vi "update file properties.vi"(4 "event name":string, 5 "mode":T2=enum."Rename Files", 6 "file format":T1(ring), 7 "scanner[]":string[](array[string]), 8 "error in":errorcluster, 9 "destination path":path, 10 "file path":path, 11 "File in":refnum<class "File.lvclass">) -> (0 "error out":errorcluster, 3 "File out":refnum<class "File.lvclass">)   [LabVIEW 2023, in "File Classes.lvlib" / "File.lvclass"]
uses:
  File.lvclass
  Controls/file operation settings mode.ctl
  File.lvclass/File.ctl
  File Classes.lvlib
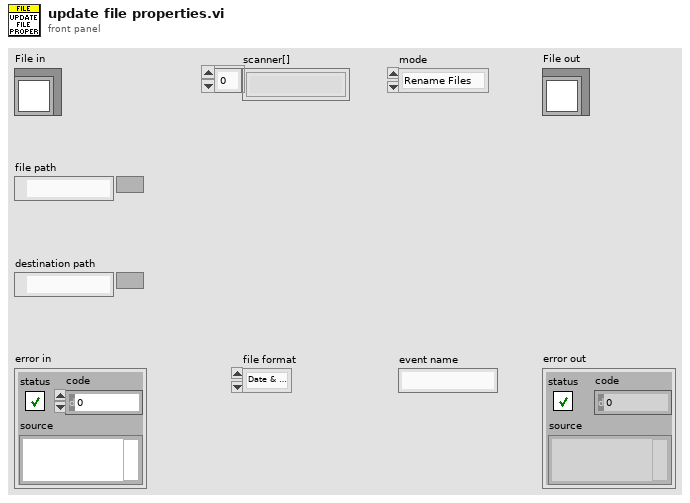
[diagram p1: front panel]
types:
  T1 = enum16{"Date & Time (Default)", "Model Sufix", "Event Sufix", "Model & Event Sufix"}
  T2 = typedef "File Classes.lvlib/file operation settings mode.ctl" = enum16{"Copy Files", "Move Files", "Rename Files"}
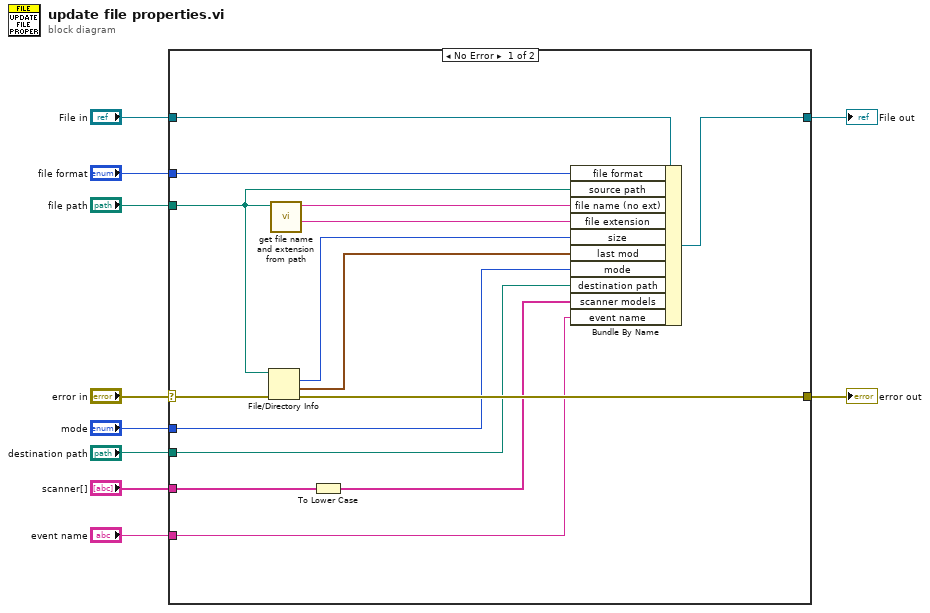
[diagram p0: block diagram]
diagram:
  n1 = case shown="No Error" "error in" {
    selector: "error in" -> [w25 w27]
    tunnel: "file path" -> [w21 _]
    tunnel: "destination path" -> [w15 _]
    tunnel: [w22 w26] -> w6
    tunnel: [w24 w27] -> w4
    tunnel: "mode" -> [w16 _]
    tunnel: "File in" -> [w23 w26]
    tunnel: "scanner[]" -> [w14 _]
    tunnel: "file format" -> [w12 _]
    tunnel: "event name" -> [w11 _]
    frame No Error {
      n2 = File/Directory Info(path=w21, error in=w25) -> (size=w18:i64, last mod=w17:timestamp, error out=w24:errorcluster)  [unwired: 4 out]
      n3 = call "get file name and extension from path.vi"("fiel path"=w21) -> ("file extension"=w19:string, "file name"=w20:string)  [unwired: 8 in, 1 out]
      n4 = To Lower Case(string=w14) -> (all lower case string=w13:string[])
      n5 = Bundle By Name(cluster=w23, "file format"=w12, "source path"=w21, "file name (no ext)"=w20, "file extension"=w19, "size"=w18, "last mod"=w17, "mode"=w16, "destination path"=w15, "scanner models"=w13, "event name"=w11) -> (w22:refnum<class "File.lvclass">)
    }
    frame Error {
    }
  }
  "error out" <- w4
  "File out" <- w6
